vi "Disable UI Controls.vi"(1 "Disable Controls?":bool, 2 "appended array":refnum<vi>[](array[refnum])) -> ()   [LabVIEW 2017]
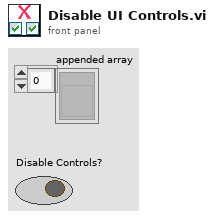
[diagram p1: front panel]
types:
  T1 = enum8{"Enabled", "Disabled", "Disabled and Grayed Out"}
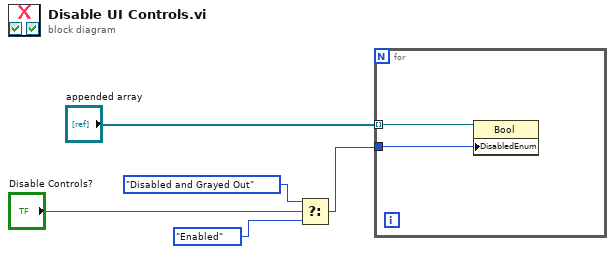
[diagram p0: block diagram]
diagram:
  n1 = Select(t=T1."Disabled and Grayed Out" ("Disabled"), s="Disable Controls?", f=T1."Enabled" ("Disabled")) -> (s? t:f=w2:T1)
  n2 = for {
    tunnel: "appended array" -> [w7] mode=indexing
    tunnel: w2 -> [w6]
    n3 = property class="Bool"(reference=w7, "DisabledEnum"=w6) -> ()  [unwired: 1 in, 2 out]
  }
